vi "Update Test Node List.vi"(8 "error in (no error)":errorcluster, 11 "Hot And Cold Source Unit View in":refnum<class "Hot And Cold Source Unit View.lvclass">) -> (0 "error out":errorcluster, 3 "Hot And Cold Source Unit View out":refnum<class "Hot And Cold Source Unit View.lvclass">)   [LabVIEW 2013, in "Hot And Cold Source Unit View.lvlib" / "Hot And Cold Source Unit View.lvclass"]
uses:
  Hot And Cold Source Unit View.lvclass
  Hot And Cold Source Unit View.lvclass/Hot And Cold Source Unit View.ctl
  Common/Control Reference/Control Reference.lvlib
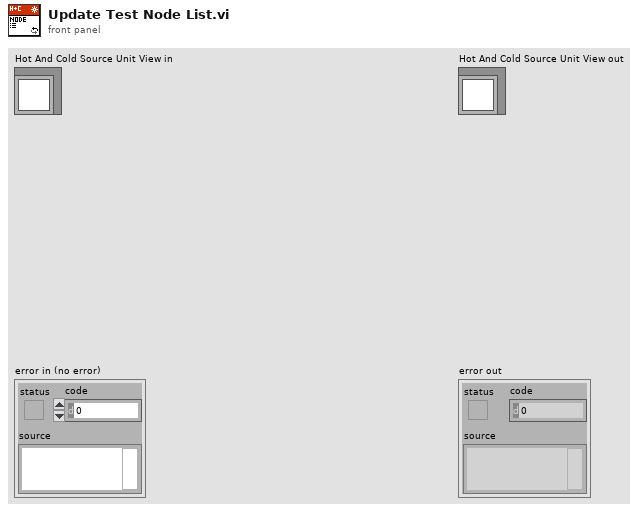
[diagram p1: front panel]
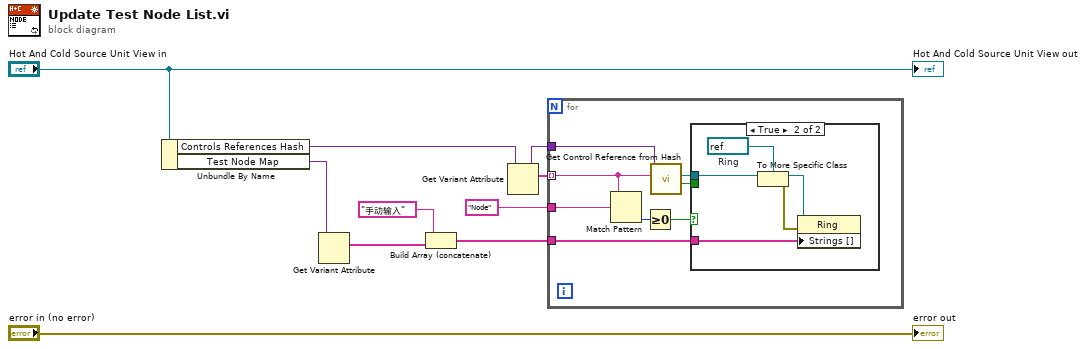
[diagram p0: block diagram]
diagram:
  n1 = Unbundle By Name("Hot And Cold Source Unit View in") -> ("Controls References Hash"=w8:variant, "Test Node Map"=w7:variant)
  n2 = Get Variant Attribute(Variant=w7) -> (names=w5:string[])  [unwired: 3 in, 3 out]
  n3 = Build Array (concatenate)("手动输入", w5) -> (w2:string[])
  n4 = Get Variant Attribute(Variant=w8) -> (duplicate Variant=w6:variant, names=w10:string[])  [unwired: 3 in, 2 out]
  n5 = for {
    tunnel: w10 -> [w17] mode=indexing
    tunnel: w6 -> [w18]
    tunnel: "Node" -> [w14]
    tunnel: w2 -> [w12]
    n6 = Match Pattern(string=w17, regular expression=w14) -> (offset past match=w15:i32)  [unwired: 1 in, 3 out]
    n7 = Greater Or Equal To 0?(x=w15) -> (x >= 0?=w13:bool)
    n8 = call "Get Control Reference from Hash.vi"("control label"=w17, "controls references hash"=w18) -> ("found?"=w11:bool, "control reference"=w16:refnum<vi>)  [unwired: 6 in, 2 out]
    n9 = case shown="True" w13 {
      tunnel: w16 -> [_ w23]
      tunnel: w12 -> [_ w20]
      tunnel: w11 -> [_ _]
      frame False {
      }
      frame True {
        w21 = refnum<vi> refnum  # Ring
        n10 = To More Specific Class(target class=w21, reference=w23) -> (specific class reference=w22:refnum<vi>, error out=w19:errorcluster)  [unwired: 1 in]
        n11 = property class="Ring"(reference=w22, error in=w19, "Strings []"=w20) -> ()  [unwired: 2 out]
      }
    }
  }
  "error out" <- "error in (no error)"
  "Hot And Cold Source Unit View out" <- "Hot And Cold Source Unit View in"
